vi "Event Handler.vi"(0 "Tamer in":refnum<class "Tamer.lvclass">, 5 "Event type":T1=enum."Message", 7 "Item Name":string, 9 "Data":variant, 11 "error in (no error)":errorcluster) -> (4 "Tamer out":refnum<class "Tamer.lvclass">, 15 "error out":errorcluster)   [LabVIEW 2020, in "Tamer.lvlib" / "Tamer.lvclass"]
doc: "This VI is the event handler of the uService: every time an event is triggered to the uService, this VI is called.\nNote: here you can access the Actor/Class data, but it will be the one coming out from Init. You cannot modify the values.\nThree different events are supported:\nI) Button Pressed: get called on a GUI button pressed. Item Name is the name (label) of the button, Data is empty.\nII) Shared Variable Updated: get called when a SV you subscribed to is updated. Item Name is the name of the SV, and Data is the value (note: you need to convert it to the proper type).\nIII) Message: get called every time a user event is generated using Send Message to Event Handler. The values of Item Name and Data are the one given to the Send Message to Event Handler.\nIV) Ready to launch?: this frame get called every time a new Run is initiated. Each uService is responsible of performing a self check before giving back the green light for the Run to start."
uses:
  Tamer.lvclass
  TALOS/TALOS_PPL.lvlibp/Father of all uServices/Father of all uServices/Event Handler Items.ctl
  Tamer Consumer Case Selector.ctl
  TALOS/TALOS_PPL.lvlibp/Support VIs/Go-NoGo.ctl
  Run Utilities/TypeDefs/Messages/Monkey Status Message.ctl
  Run Utilities/TypeDefs/Monkey Status.ctl
  Run Utilities/Schedule/Schedule.lvclass
  Run Utilities/TypeDefs/Messages/Script Checker Message.ctl
  Run Utilities/TypeDefs/Script Checker Result.ctl
  Run Utilities/TypeDefs/Messages/Banana Message.ctl
  Run Utilities/TypeDefs/Return Code.ctl
  Tamer.lvclass/Tamer.ctl
  TALOS/TALOS_PPL.lvlibp/Guardian/Guardian/Requests.ctl
  Open Debug Window.vi
  TALOS/TALOS_PPL.lvlibp/Father of all uServices/Father of all uServices/Father of all uServices.lvclass
  TALOS/TALOS_PPL.lvlibp
  TALOS/TALOS_PPL.lvlibp/Guardian/Guardian/Guardian.lvclass
  Run Utilities/Run Utilities.lvlib
  C:/LabVIEW Code/aegis-labview-code/TALOS/TALOS_PPL.lvlibp/Father of all uServices/Father of all uServices/Father of all uServices.lvclass
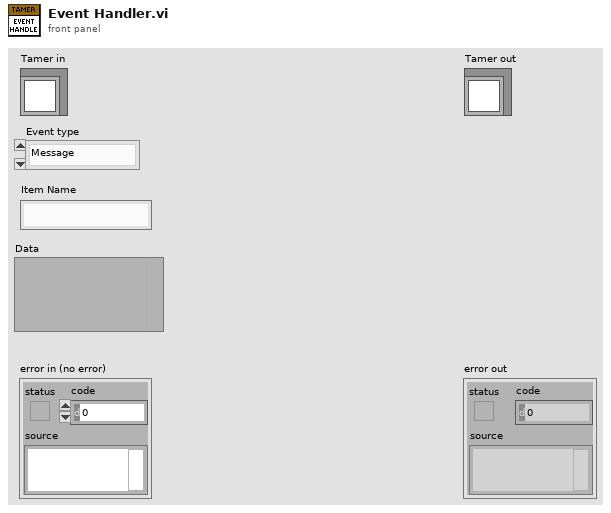
[diagram p1: front panel]
types:
  T1 = typedef "TALOS_PPL.lvlibp/Father of all uServices.lvlib/Father of all uServices.lvclass/Event Handler Items.ctl" = enum16{"Button Pressed", "Message", "Ready to launch?", "Safe Mode", "Start RUN", "Stop RUN"}
  T2 = typedef "Tamer.lvlib/Tamer.lvclass/Tamer Consumer Case Selector.ctl" = enum16{"New schedule", "Initiate RUN", "Parse Schedules", "Script Checker", "Banana after Quality Check", "Update Crit Lvl", "Propagate Banana", "Reply from Guardian", "Reply from uService", "Timeout of RUN", "uService Replies Check", "Update from Monkey", "Monkey Died", "Reschedule", "Rerun", "Stop DAQ", "Stop Schedule", "Skip Run", "Kill Process", "Update GV"}
  T3 = enum32{"Invalid", "Standard", "Closed", "Hidden", "Minimized", "Maximized"}
  T4 = typedef "TALOS_PPL.lvlibp/Go-NoGo.ctl" = cluster{"ID":string, "Status":bool, "Data":string[], "GUID":string}
  T5 = typedef "Run Utilities.lvlib/Monkey Status Message.ctl" = cluster{"Monkey ID":string, "Monkey Status":T6, "Scripts left":u32, "ETA":string, "Current Action":string, "Report from previous RUNs":string, "Skipped RUNs":refnum<class "Schedule.lvclass">}
  T6 = typedef "Run Utilities.lvlib/Monkey Status.ctl" = enum16{"Init", "Paused", "Ongoing", "Stopped", "Finished (no errors)", "Finished (with errors)"}
  T7 = typedef "Run Utilities.lvlib/Script Checker Message.ctl" = cluster{"Monkey ID":string, "Script Checker Result":T8}
  T8 = typedef "Run Utilities.lvlib/Script Checker Result.ctl" = enum16{"Passed", "Failed", "Empty"}
  T9 = typedef "Run Utilities.lvlib/Return Code.ctl" = enum16{"All Good", "Retry", "Skip", "Skip All", "ABORT"}
  T10 = typedef "Run Utilities.lvlib/Banana Message.ctl" = cluster{"FPGA Name":string, "Return Code":T9}
  T11 = typedef "TALOS_PPL.lvlibp/Guardian.lvlib/Guardian.lvclass/Requests.ctl" = enum16{"Ready to Launch", "Start RUN", "Stop RUN", "Update DAQ Params", "Update Error Listbox", "Update Run Status", "Update Kasli Log", "Run Stopped with Errors", "Switch uS View"}
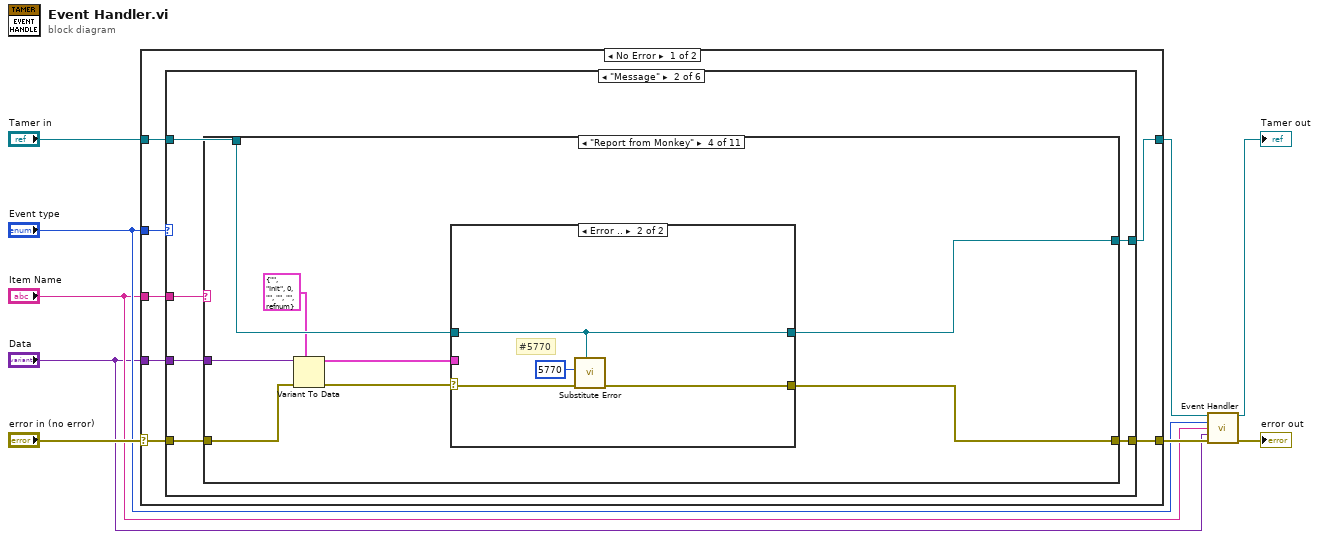
[diagram p0: block diagram]
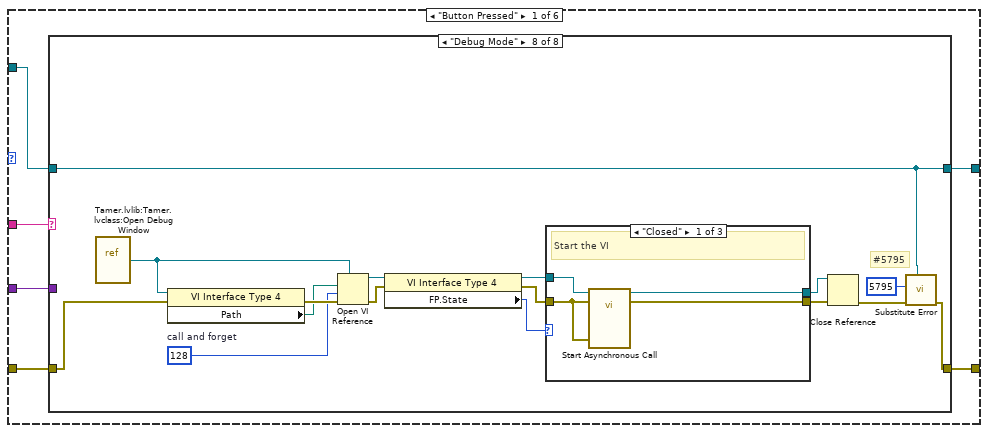
[diagram p2: hidden frame]
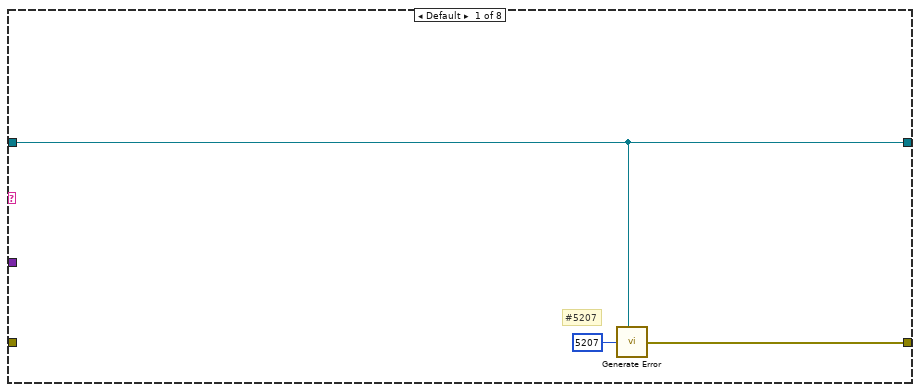
[diagram p3: hidden frame]
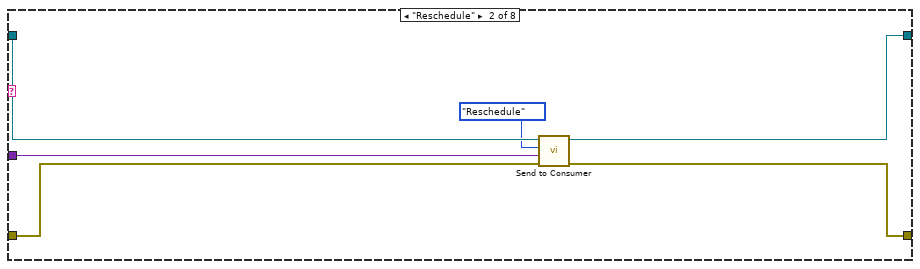
[diagram p4: hidden frame]
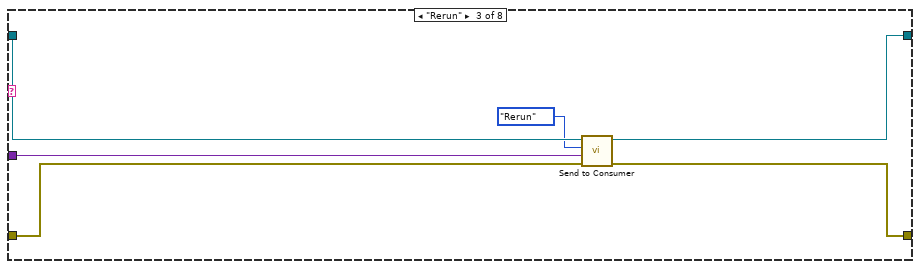
[diagram p5: hidden frame]
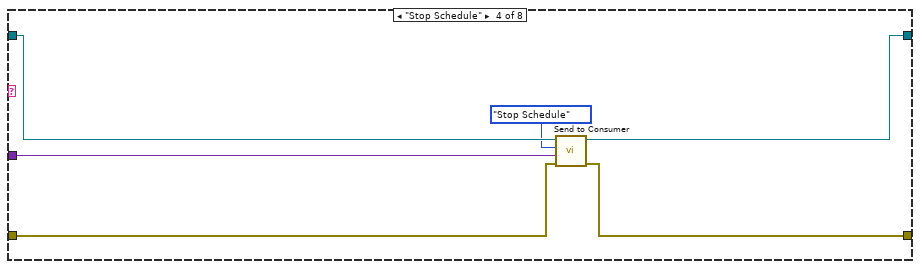
[diagram p6: hidden frame]
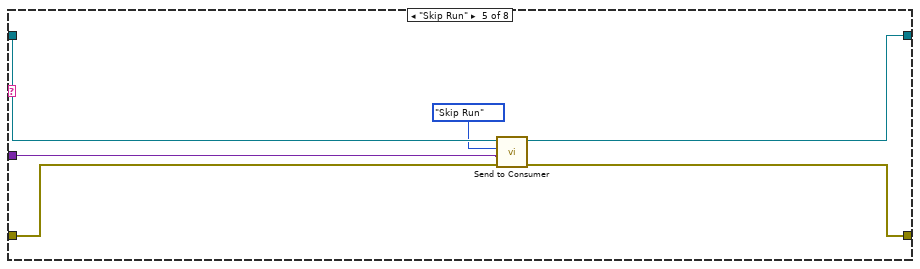
[diagram p7: hidden frame]
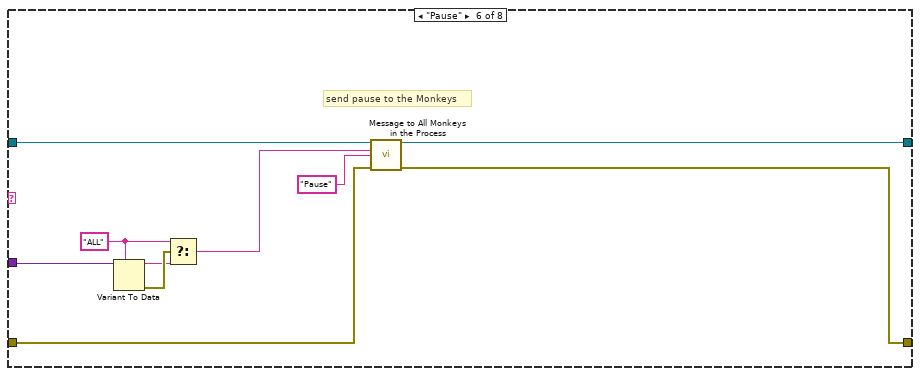
[diagram p8: hidden frame]
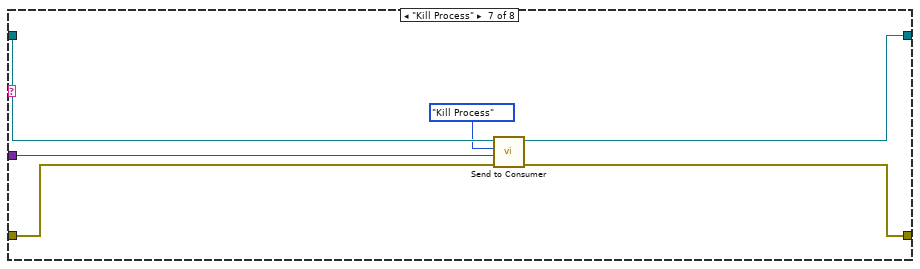
[diagram p9: hidden frame]
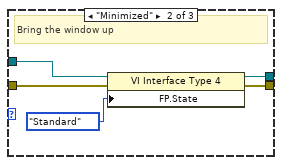
[diagram p10: hidden frame]
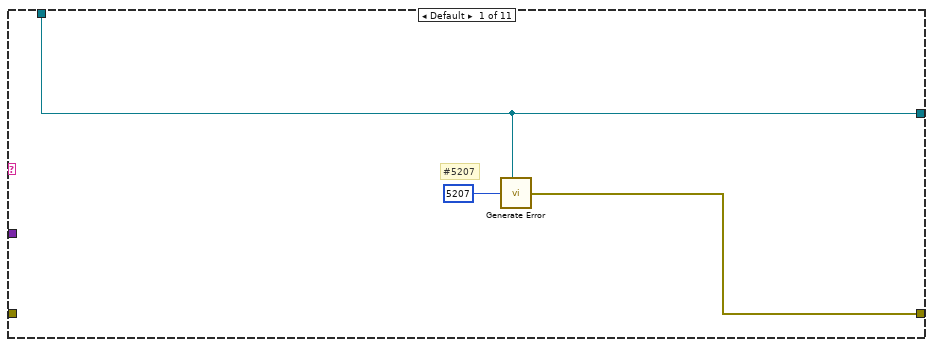
[diagram p12: hidden frame]
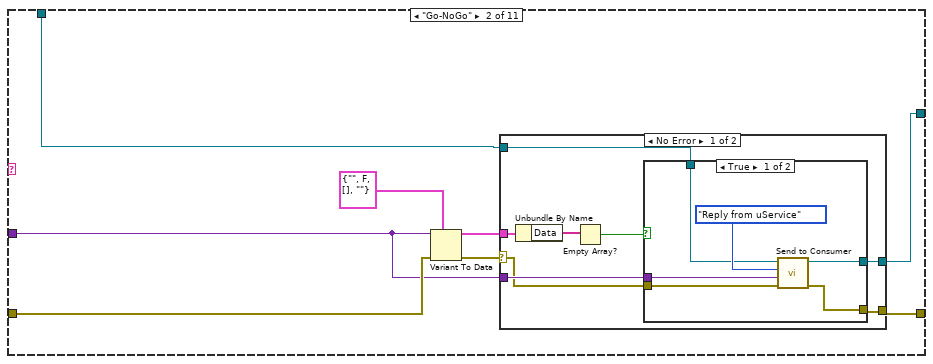
[diagram p13: hidden frame]
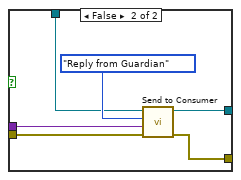
[diagram p14: hidden frame]
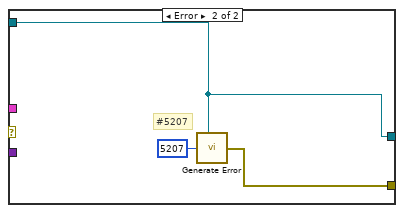
[diagram p15: hidden frame]
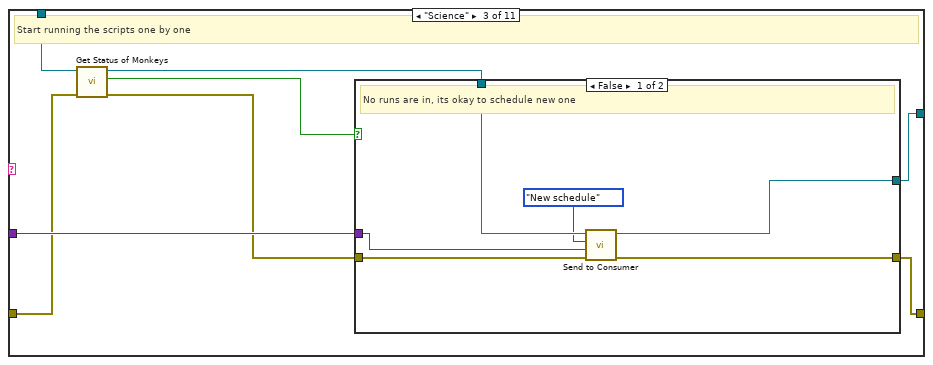
[diagram p16: hidden frame]
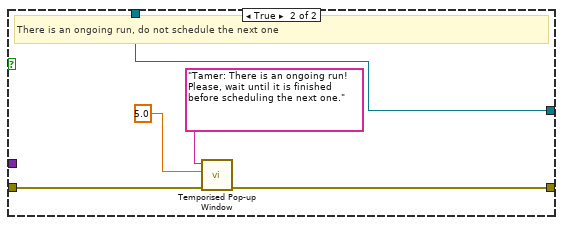
[diagram p17: hidden frame]
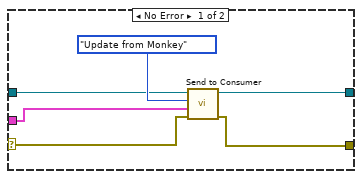
[diagram p18: hidden frame]
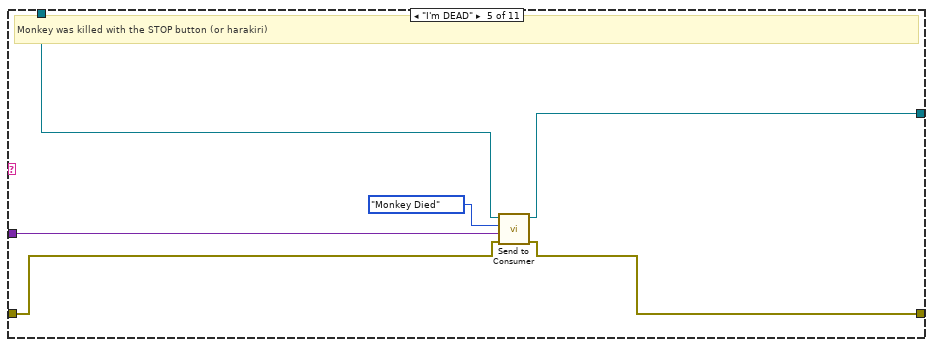
[diagram p19: hidden frame]
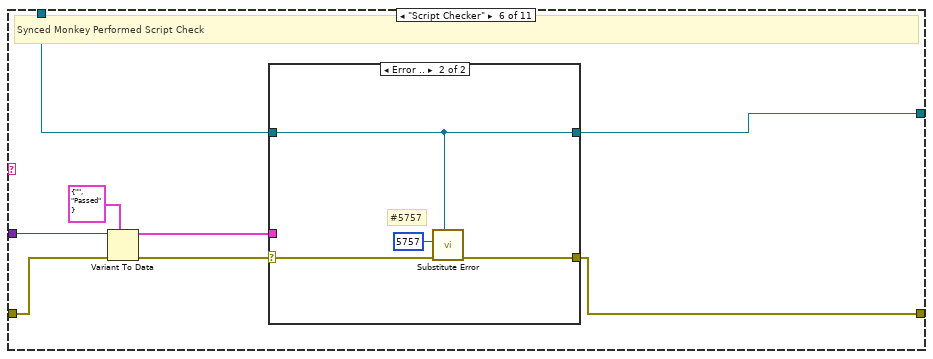
[diagram p20: hidden frame]
diagram:
  n1 = case shown="No Error" "error in (no error)" {
    selector: "error in (no error)" -> [w14 w328]
    tunnel: [w15 w328] -> w7
    tunnel: [w11 w327] -> w4
    tunnel: "Tamer in" -> [w10 w327]
    tunnel: "Event type" -> [w16 _]
    tunnel: "Item Name" -> [w13 _]
    tunnel: "Data" -> [w12 _]
    frame No Error {
      n2 = case shown="\"Message\"" w16 {
        tunnel: [w22 w94 w305 w314 w319 w326] -> w15
        tunnel: w14 -> [w19 w98 w306 w316 w320 w324]
        tunnel: w13 -> [w20 w97 _ _ _ _]
        tunnel: w10 -> [w21 w95 w304 w311 w321 w325]
        tunnel: w12 -> [w17 w96 w302 _ _ _]
        tunnel: [w18 w93 w301 w313 w317 w322] -> w11
        frame "Button Pressed" {
          n3 = case shown="\"Debug Mode\"" w20 {
            tunnel: w19 -> [_ w26 w32 w39 w45 w56 w63 w77]
            tunnel: [w24 w30 w35 w42 w46 w55 w60 w66] -> w22
            tunnel: w21 -> [w23 w31 w37 w43 w49 w58 w65 w67]
            tunnel: [w23 w28 w34 w41 w47 w57 w61 w67] -> w18
            tunnel: w17 -> [_ w27 w33 w38 w44 w54 w62 _]
            frame Default {
              # "#5207"
              n4 = call "Generate Error.vi"("Class"=w23, "Error Code"=5207) -> ("error out"=w24:errorcluster)  [unwired: 5 in]
            }
            frame "Reschedule" {
              n5 = call "Send to Consumer.vi"("error in (no error)"=w26, "Data"=w27, "Case ID"=Tamer_Consumer_Case_Selector."Reschedule" ("Monkey Consumer Case Selector"), "uService Template in"=w31) -> ("error out"=w30:errorcluster, "uService Template out"=w28:refnum<class "Tamer.lvclass">)  [unwired: 6 in]
            }
            frame "Rerun" {
              n6 = call "Send to Consumer.vi"("error in (no error)"=w32, "Data"=w33, "Case ID"=Tamer_Consumer_Case_Selector."Rerun" ("Monkey Consumer Case Selector"), "uService Template in"=w37) -> ("error out"=w35:errorcluster, "uService Template out"=w34:refnum<class "Tamer.lvclass">)  [unwired: 6 in]
            }
            frame "Stop Schedule" {
              n7 = call "Send to Consumer.vi"("error in (no error)"=w39, "Data"=w38, "Case ID"=Tamer_Consumer_Case_Selector."Stop Schedule" ("Monkey Consumer Case Selector"), "uService Template in"=w43) -> ("error out"=w42:errorcluster, "uService Template out"=w41:refnum<class "Tamer.lvclass">)  [unwired: 6 in]
            }
            frame "Skip Run" {
              n8 = call "Send to Consumer.vi"("error in (no error)"=w45, "Data"=w44, "Case ID"=Tamer_Consumer_Case_Selector."Skip Run" ("Monkey Consumer Case Selector"), "uService Template in"=w49) -> ("error out"=w46:errorcluster, "uService Template out"=w47:refnum<class "Tamer.lvclass">)  [unwired: 6 in]
            }
            frame "Pause" {
              w53 = "ALL"
              # "send pause to the Monkeys"
              n9 = Variant To Data(type=w53, Variant=w54) -> (data=w52:string, error out=w59:errorcluster)  [unwired: 1 in]
              n10 = Select(t=w53, s=w59, f=w52) -> (s? t:f=w51:string)
              n11 = call-dynamic "Message to All Monkeys in the Process.vi"("Tamer in"=w58, "Process ID"=w51, "Message"="Pause" ("Process ID"), "error in (no error)"=w56) -> ("Tamer out"=w57:refnum<class "Tamer.lvclass">, "error out"=w55:errorcluster)  [unwired: 10 in]
            }
            frame "Kill Process" {
              n12 = call "Send to Consumer.vi"("error in (no error)"=w63, "Data"=w62, "Case ID"=Tamer_Consumer_Case_Selector."Kill Process" ("Monkey Consumer Case Selector"), "uService Template in"=w65) -> ("error out"=w60:errorcluster, "uService Template out"=w61:refnum<class "Tamer.lvclass">)  [unwired: 6 in]
            }
            frame "Debug Mode" {
              w78 = 128  # call and forget
              # "#5795"
              n13 = vi-ref "Tamer.lvlib:Tamer.lvclass:Open Debug Window.vi"() -> (w76:refnum<vi>)
              n14 = property class="VI Interface Type 4"(reference=w76, error in=w77) -> (error out=w81:errorcluster, "Path"=w80:path)  [unwired: 1 out]
              n15 = Open VI Reference(type specifier VI Refnum (for type only)=w76, vi path=w80, options=w78, error in (no error)=w81) -> (vi reference=w79:refnum<vi>, error out=w74:errorcluster)  [unwired: 2 in]
              n16 = property class="VI Interface Type 4"(reference=w79, error in=w74) -> (reference out=w75:refnum<vi>, error out=w73:errorcluster, "FP.State"=w72:T3)
              n17 = case shown="\"Closed\"" w72 {
                tunnel: w75 -> [w85 w88 w92]
                tunnel: w73 -> [w84 w90 w91]
                tunnel: [w83 w89 w91] -> w69
                tunnel: [w82 w86 w92] -> w68
                frame "Closed" {
                  # "Start the VI"
                  n18 = call-by-ref "Start Asynchronous Call"(reference=w85, error in=w84, 8:"error in (no error)"=w84) -> (reference out=w82:refnum<vi>, error out=w83:errorcluster)  [unwired: 10 in, 1 out]
                }
                frame "Minimized" {
                  # "Bring the window up"
                  n19 = property class="VI Interface Type 4"(reference=w88, error in=w90, "FP.State"=T3."Standard" ("Front Panel Window:State")) -> (reference out=w86:refnum<vi>, error out=w89:errorcluster)
                }
                frame Default {
                  # "Either running or something is worng, do nothing"
                }
              }
              n20 = Close Reference(reference=w68, error in (no error)=w69) -> (error out=w71:errorcluster)
              n21 = call "Substitute Error.vi"("LabVIEW Object"=w67, "error in (no error)"=w71, "Error Code"=5795) -> ("error out"=w66:errorcluster)  [unwired: 8 in]
            }
          }
        }
        frame "Message" {
          n22 = case shown="\"Report from Monkey\"" w97 {
            tunnel: w98 -> [_ w108 w138 w158 w171 w182 w199 w237 w257 w274 w291]
            tunnel: w96 -> [_ w105 w140 w159 w172 w181 w201 w233 w256 w279 _]
            tunnel: w95 -> [w99 w103 w137 w156 w175 w178 w195 w238 w255 w276 w288]
            tunnel: [w100 w109 w139 w153 w174 w176 w196 w234 w258 w269 w290] -> w94
            tunnel: [w99 w102 w133 w152 w170 w177 w194 w243 w254 w277 w289] -> w93
            frame Default {
              # "#5207"
              n23 = call "Generate Error.vi"("Class"=w99, "Error Code"=5207) -> ("error out"=w100:errorcluster)  [unwired: 5 in]
            }
            frame "Go-NoGo" {
              n24 = Variant To Data(error in=w108, type=T4 {"ID"="", "Status"=FALSE, "Data"=[], "GUID"=""} ("Go-NoGo"), Variant=w105) -> (data=w104:T4, error out=w106:errorcluster)
              n25 = case shown="No Error" w106 {
                selector: w106 -> [w112 _]
                tunnel: [w117 w131] -> w109
                tunnel: w105 -> [w116 _]
                tunnel: w104 -> [w115 _]
                tunnel: w103 -> [w111 w130]
                tunnel: [w110 w130] -> w102
                frame No Error {
                  n26 = Unbundle By Name(w115) -> ("Data"=w114:string[])
                  n27 = Empty Array?(array=w114) -> (empty?=w113:bool)
                  n28 = case shown="True" w113 {
                    tunnel: [w123 w129] -> w117
                    tunnel: w116 -> [w121 w127]
                    tunnel: w112 -> [w120 w126]
                    tunnel: w111 -> [w119 w125]
                    tunnel: [w118 w124] -> w110
                    frame True {
                      n29 = call "Send to Consumer.vi"("error in (no error)"=w120, "Data"=w121, "Case ID"=Tamer_Consumer_Case_Selector."Reply from uService" ("Monkey Consumer Case Selector"), "uService Template in"=w119) -> ("error out"=w123:errorcluster, "uService Template out"=w118:refnum<class "Tamer.lvclass">)  [unwired: 6 in]
                    }
                    frame False {
                      n30 = call "Send to Consumer.vi"("error in (no error)"=w126, "Data"=w127, "Case ID"=Tamer_Consumer_Case_Selector."Reply from Guardian" ("Monkey Consumer Case Selector"), "uService Template in"=w125) -> ("error out"=w129:errorcluster, "uService Template out"=w124:refnum<class "Tamer.lvclass">)  [unwired: 6 in]
                    }
                  }
                }
                frame Error {
                  # "#5207"
                  n31 = call "Generate Error.vi"("Class"=w130, "Error Code"=5207) -> ("error out"=w131:errorcluster)  [unwired: 5 in]
                }
              }
            }
            frame "Science" {
              # "Start running the scripts one by one"
              n32 = call-dynamic "Get Status of Monkeys.vi"("error in (no error)"=w138, "Tamer in"=w137) -> ("error out"=w135:errorcluster, "Anything running?"=w134:bool, "Tamer out"=w136:refnum<class "Tamer.lvclass">)  [unwired: 7 in]
              n33 = case shown="False" w134 {
                tunnel: w140 -> [w143 _]
                tunnel: [w146 w148] -> w139
                tunnel: w136 -> [w145 w147]
                tunnel: w135 -> [w142 w151]
                tunnel: [w141 w147] -> w133
                frame False {
                  # "No runs are in, its okay to schedule new one"
                  n34 = call "Send to Consumer.vi"("error in (no error)"=w142, "Data"=w143, "Case ID"=Tamer_Consumer_Case_Selector."New schedule" ("Monkey Consumer Case Selector"), "uService Template in"=w145) -> ("error out"=w146:errorcluster, "uService Template out"=w141:refnum<class "Tamer.lvclass">)  [unwired: 6 in]
                }
                frame True {
                  # "There is an ongoing run, do not schedule the next one"
                  n35 = call "Temporised Pop-up Window.vi"("error in (no error)"=w151, "Timeout"=5.0, "Text"="Tamer: There is an ongoing run! Please, wait until it is finished before scheduling the next one.") -> ("error out"=w148:errorcluster)  [unwired: 8 in]
                }
              }
            }
            frame "Report from Monkey" {
              n36 = Variant To Data(error in=w158, type=T5 {"Monkey ID"="", "Monkey Status"=enum."Init", "Scripts left"=0, "ETA"="", "Current Action"="", "Report from previous RUNs"="", "Skipped RUNs"=refnum} ("Monkey Status Message"), Variant=w159) -> (data=w155:T5, error out=w157:errorcluster)
              n37 = case shown="Error .." w157 {
                selector: w157 -> [w164 w169]
                tunnel: w156 -> [w163 w166]
                tunnel: w155 -> [w162 _]
                tunnel: [w161 w167] -> w153
                tunnel: [w160 w166] -> w152
                frame No Error {
                  n38 = call "Send to Consumer.vi"("error in (no error)"=w164, "Data"=w162, "Case ID"=Tamer_Consumer_Case_Selector."Update from Monkey" ("Monkey Consumer Case Selector"), "uService Template in"=w163) -> ("error out"=w161:errorcluster, "uService Template out"=w160:refnum<class "Tamer.lvclass">)  [unwired: 6 in]
                }
                frame Error {
                  # "#5770"
                  n39 = call "Substitute Error.vi"("LabVIEW Object"=w166, "error in (no error)"=w169, "Error Code"=5770) -> ("error out"=w167:errorcluster)  [unwired: 8 in]
                }
              }
            }
            frame "I'm DEAD" {
              # "Monkey was killed with the STOP button (or harakiri)"
              n40 = call "Send to Consumer.vi"("error in (no error)"=w171, "Data"=w172, "Case ID"=Tamer_Consumer_Case_Selector."Monkey Died" ("Monkey Consumer Case Selector"), "uService Template in"=w175) -> ("error out"=w174:errorcluster, "uService Template out"=w170:refnum<class "Tamer.lvclass">)  [unwired: 6 in]
            }
            frame "Script Checker" {
              # "Synced Monkey Performed Script Check"
              n41 = Variant To Data(error in=w182, type=T7 {"Monkey ID"="", "Script Checker Result"=enum."Passed"} ("Message"), Variant=w181) -> (data=w179:T7, error out=w180:errorcluster)
              n42 = case shown="Error .." w180 {
                selector: w180 -> [w185 w191]
                tunnel: [w189 w192] -> w176
                tunnel: w178 -> [w188 w190]
                tunnel: w179 -> [w187 _]
                tunnel: [w184 w190] -> w177
                frame No Error {
                  n43 = call "Send to Consumer.vi"("error in (no error)"=w185, "Data"=w187, "Case ID"=Tamer_Consumer_Case_Selector."Script Checker" ("Monkey Consumer Case Selector"), "uService Template in"=w188) -> ("error out"=w189:errorcluster, "uService Template out"=w184:refnum<class "Tamer.lvclass">)  [unwired: 6 in]
                }
                frame Error {
                  # "#5757"
                  n44 = call "Substitute Error.vi"("LabVIEW Object"=w190, "error in (no error)"=w191, "Error Code"=5757) -> ("error out"=w192:errorcluster)  [unwired: 8 in]
                }
              }
            }
            frame "B4n4n4" {
              # "Script finished. Send it to Monkey for the quality check"
              n45 = Variant To Data(error in=w199, type=string[] [], Variant=w201) -> (data=w198:string[], error out=w197:errorcluster)
              n46 = case shown="No Error" w197 {
                selector: w197 -> [w224 w232]
                tunnel: w198 -> [w228 _]
                tunnel: [w208 w231] -> w196
                tunnel: w195 -> [w222 w229]
                tunnel: [w219 w229] -> w194
                frame No Error {
                  w202 = "Quality Check" ("Message")
                  # "#5752\nB4n4n4"
                  n47 = Index Array(array=w228) -> (element #1=w209:string, element #2=w225:string)  [unwired: 2 in]
                  n48 = Decimal String To Number(string=w225, default (0L)=3) -> (number=w226:i32)  [unwired: 1 in, 1 out]
                  n49 = Variant To Data(error in=w224, type=Return_Code."Skip All" ("Return Code"), Variant=w226) -> (data=w218:T9, error out=w221:errorcluster)
                  n50 = call-dynamic "Get Monkey ID From FPGA Name.vi"("error in (no error)"=w221, "FPGA Name"=w209, "Tamer in"=w222) -> ("error out"=w217:errorcluster, "Monkey ID"=w212:string, "Tamer out"=w216:refnum<class "Tamer.lvclass">)  [unwired: 6 in]
                  n51 = Bundle(cluster=T10 {"FPGA Name"="", "Return Code"=enum."All Good"} ("Cluster"), "FPGA Name"=w209, "Return Code"=w218) -> (w207:T10)
                  n52 = call "Message to uService.vi"("Father of all uServices in"=w216, "uService ID"=w212, "Message"=w202, "Data"=w207, "error in (no error)"=w217) -> ("Father of all uServices out"=w206:refnum<class "Tamer.lvclass">, "error out"=w213:errorcluster)  [unwired: 9 in]
                  n53 = Concatenate Strings(w202, " to " ("string"), w212) -> (w211:string)
                  n54 = call "FPGA informative error on return.vi"("Message"=w207, "Class in"=w206) -> ("error out"=w204:errorcluster)  [unwired: 9 in]
                  n55 = call-dynamic "Update Action History.vi"("error in (no error)"=w213, "Action"=w211, "Tamer in"=w206) -> ("error out"=w205:errorcluster, "Tamer out"=w219:refnum<class "Tamer.lvclass">)  [unwired: 7 in]
                  n56 = Merge Errors(w205, w204) -> (w203:errorcluster)
                  n57 = call "Substitute Error.vi"("LabVIEW Object"=w219, "error in (no error)"=w203, "Error Code"=5752, "Optional String"="Tamer doesn't know who sent B4n4n4") -> ("error out"=w208:errorcluster)  [unwired: 7 in]
                }
                frame Error {
                  # "#5789"
                  n58 = call "Substitute Error.vi"("LabVIEW Object"=w229, "error in (no error)"=w232, "Error Code"=5789) -> ("error out"=w231:errorcluster)  [unwired: 8 in]
                }
              }
            }
            frame "Quality Check - result" {
              n59 = Variant To Data(type=T10 {"FPGA Name"="", "Return Code"=enum."All Good"} ("Cluster"), Variant=w233) -> (data=w239:T10, error out=w240:errorcluster)  [unwired: 1 in]
              n60 = case shown="No Error" w240 {
                tunnel: w239 -> [w248 _]
                tunnel: w238 -> [w251 w252]
                tunnel: [w246 _] -> w235
                tunnel: [w247 w252] -> w244
                frame No Error {
                  # "Check if quality of run was passed. If not, give an error to have that information in the error log"
                  n61 = Unbundle By Name(w248) -> ("FPGA Name"=w249:string)
                  n62 = Concatenate Strings("Received the quality check from ", w249) -> (w245:string)
                  n63 = call-dynamic "Update Action History.vi"("Action"=w245, "Tamer in"=w251) -> ("error out"=w246:errorcluster, "Tamer out"=w247:refnum<class "Tamer.lvclass">)  [unwired: 8 in]
                }
                frame Error {
                  # "Wrong format, this is delt with in the consumer"
                }
              }
              n64 = call "Send to Consumer.vi"("error in (no error)"=w237, "Data"=w233, "Case ID"=Tamer_Consumer_Case_Selector."Banana after Quality Check" ("Monkey Consumer Case Selector"), "uService Template in"=w244) -> ("error out"=w236:errorcluster, "uService Template out"=w243:refnum<class "Tamer.lvclass">)  [unwired: 6 in]
              n65 = Merge Errors(w236, w235) -> (w234:errorcluster)
            }
            frame "570prun" {
              # "True= StartRun given, False = StopRun given"
              # "Issue Stop Run to all the uServices and Guardians."
              n66 = Unbundle By Name(w255) -> ("StartRun/StopRun toggle"=w253:bool)
              n67 = case shown="True" w253 {
                tunnel: [w260 w268] -> w258
                tunnel: w257 -> [w260 w267]
                tunnel: w256 -> [_ w266]
                tunnel: w255 -> [w259 w264]
                tunnel: [w259 w262] -> w254
                frame False {
                  # "Do nothing"
                }
                frame True {
                  # "#STOP_RUN"
                  n68 = call "Request to Guardian.vi"("error in (no error)"=w267, "Data"=w266, "Requests"=Requests."Stop RUN", "Father of all uServices in"=w264) -> ("error out"=w268:errorcluster, "Father of all uServices out"=w263:refnum<class "Tamer.lvclass">)  [unwired: 6 in]
                  n69 = Bundle By Name(cluster=w263, "StartRun/StopRun toggle"=FALSE) -> (w262:refnum<class "Tamer.lvclass">)
                }
              }
            }
            frame "Error Criticality" {
              # "Error occured when running a script"
              n70 = call-dynamic "Get Status of Monkeys.vi"("error in (no error)"=w274, "Tamer in"=w276) -> ("error out"=w280:errorcluster, "Anything running?"=w272:bool, "Tamer out"=w275:refnum<class "Tamer.lvclass">)  [unwired: 7 in]
              n71 = Not(x=w280) -> (.not. x?=w273:bool)
              n72 = Select(t=w272, s=w273, f=TRUE) -> (s? t:f=w270:bool)
              n73 = case shown="True" w270 {
                tunnel: w279 -> [_ w285]
                tunnel: [_ w284] -> w278
                tunnel: [w281 w282] -> w277
                tunnel: w275 -> [w281 w286]
                frame False {
                }
                frame True {
                  n74 = call "Send to Consumer.vi"("Data"=w285, "Case ID"=Tamer_Consumer_Case_Selector."Update Crit Lvl" ("Monkey Consumer Case Selector"), "uService Template in"=w286) -> ("error out"=w284:errorcluster, "uService Template out"=w282:refnum<class "Tamer.lvclass">)  [unwired: 7 in]
                }
              }
              n75 = Merge Errors(w278, w280) -> (w269:errorcluster)
            }
            frame "5cr47ch_y0ur_h34d" {
              # "True= StartRun given, False = StopRun given"
              # "Start the Run, but only if wasn't already started"
              n76 = Unbundle By Name(w288) -> ("StartRun/StopRun toggle"=w287:bool)
              n77 = case shown="False" w287 {
                tunnel: w291 -> [w298 w299]
                tunnel: [w297 w299] -> w290
                tunnel: [w294 w300] -> w289
                tunnel: w288 -> [w292 w300]
                frame False {
                  # "#START_RUN"
                  n78 = call "Request to Guardian.vi"("error in (no error)"=w298, "Requests"=Requests."Start RUN", "Father of all uServices in"=w292) -> ("error out"=w297:errorcluster, "Father of all uServices out"=w296:refnum<class "Tamer.lvclass">)  [unwired: 7 in]
                  n79 = Bundle By Name(cluster=w296, "StartRun/StopRun toggle"=TRUE ("StartRun already given?")) -> (w294:refnum<class "Tamer.lvclass">)
                }
                frame True {
                  # "Do nothing"
                }
              }
            }
          }
        }
        frame "Ready to launch?" {
          # "Don't remove this wire!"
          # "Just give green light: \"Cogito ergo sum\" - Volpe"
          n80 = call-dynamic "Go-NoGo.vi"("error in (no error)"=w306, "Go-NoGo Data"=w302, "Go?"=TRUE, "Father of all uServices in"=w304) -> ("error out"=w305:errorcluster, "Father of all uServices out"=w301:refnum<class "Tamer.lvclass">)  [unwired: 6 in]
        }
        frame "Safe Mode" {
          n81 = call-dynamic "Update Monkeys Status.vi"("In ALL?"=TRUE, "Status"=Monkey_Status."Finished (with errors)", "Tamer in"=w311) -> ("error out"=w309:errorcluster, "Tamer out"=w312:refnum<class "Tamer.lvclass">)  [unwired: 7 in]
          n82 = call "Send to Consumer.vi"("Case ID"=Tamer_Consumer_Case_Selector."Stop Schedule" ("Monkey Consumer Case Selector"), "uService Template in"=w312) -> ("error out"=w310:errorcluster, "uService Template out"=w313:refnum<class "Tamer.lvclass">)  [unwired: 8 in]
          n83 = Merge Errors(w310, w309, w316) -> (w314:errorcluster)
        }
        frame "Start RUN" {
          n84 = call-dynamic "Update Action History.vi"("error in (no error)"=w320, "Action"="Start Run" ("GUI Item Name"), "Tamer in"=w321) -> ("error out"=w319:errorcluster, "Tamer out"=w317:refnum<class "Tamer.lvclass">)  [unwired: 7 in]
        }
        frame "Stop RUN" {
          n85 = call-dynamic "Update Action History.vi"("error in (no error)"=w324, "Action"="Experiment finished! Ending the script..." ("GUI Item Name"), "Tamer in"=w325) -> ("error out"=w326:errorcluster, "Tamer out"=w322:refnum<class "Tamer.lvclass">)  [unwired: 7 in]
        }
      }
    }
    frame Error {
    }
  }
  n86 = call-parent "Event Handler.vi"("uService Template in"=w4, "Event type"="Event type", "Item Name"="Item Name", "Data"="Data", "error in (no error)"=w7) -> ("uService Template out"=→"Tamer out":refnum<class "Tamer.lvclass">, "error out"=→"error out":errorcluster)  [unwired: 9 in]
